vi "DFD Integer Delay with State (Array).vi"(6 "state in":dbl[](array[numeric]), 8 "error in (no error)":errorcluster, 10 "delay":i32=1, 11 "signal in":dbl[](array[numeric])) -> (0 "error out":errorcluster, 3 "signal out":dbl[](array[numeric]), 4 "state out":dbl[](array[numeric]))   [LabVIEW 2017, in "NI_DigFilterLicensed.lvlib"]
doc: "Delays a signal by a specified integer number of sample intervals. You must specify the initial internal states in the <B>state in</B> input to generate an accurate output. Wire data to the <B>signal in</B> input to determine the polymorphic instance to use or manually select the instance."
uses:
  <vilib>/addons/Digital Filter Design/NI_DigFilterLicensed.lvlib
  <vilib>/addons/Digital Filter Design/NI_DigFilter_Process.lvlib
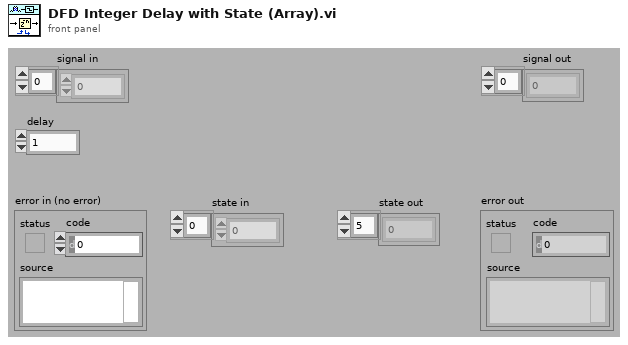
[diagram p1: front panel]
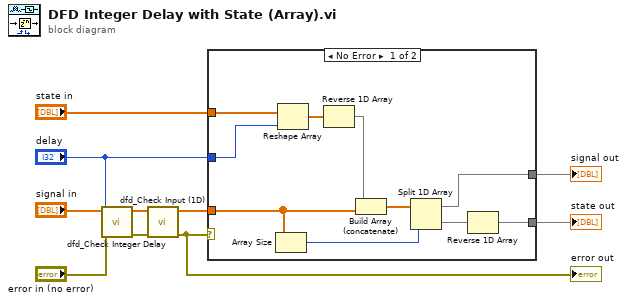
[diagram p0: block diagram]
diagram:
  n1 = call <vilib>:"dfd_Check Integer Delay.vi"("error in (no error)"="error in (no error)", "delay in"="delay") -> ("error out"=w5:errorcluster)  [unwired: 9 out]
  n2 = call <vilib>:"dfd_Check Input (1D).vi"("error in (no error)"=w5, "x"="signal in") -> ("error out"=w1:errorcluster, "dup x"=w2:dbl[])  [unwired: 1 in, 7 out]
  "error out" <- w1
  n3 = case shown="No Error" w1 {
    tunnel: "state in" -> [w19 _]
    tunnel: "delay" -> [w17 _]
    tunnel: [w10 _] -> w8
    tunnel: [w18 _] -> w7
    tunnel: w2 -> [w16 _]
    frame No Error {
      n4 = Array Size(array=w16) -> (size(s)=w11:i32)
      n5 = Reshape Array(w19, w17) -> (w15:dbl[])
      n6 = Reverse 1D Array(array=w15) -> (reversed array=w14:dbl[])
      n7 = Build Array (concatenate)(w14, w16) -> (w13:dbl[])
      n8 = Split 1D Array(array=w13, index=w11) -> (first subarray=w10:dbl[], second subarray=w12:dbl[])
      n9 = Reverse 1D Array(array=w12) -> (reversed array=w18:dbl[])
    }
    frame Error {
    }
  }
  "signal out" <- w8
  "state out" <- w7
